vi "Net DC Global Gain Update.vi"(4 "Global Gain Correction":dbl, 5 "Device Trim List":string) -> (2 "Updated Trim List":string)   [LabVIEW 2010]
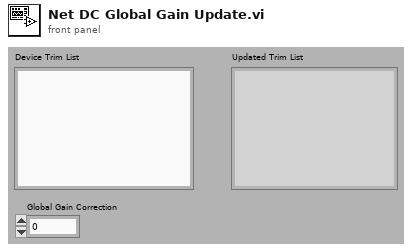
[diagram p1: front panel]
types:
  T1 = enum16{"U8", "U16", "U32", "U64", "I8", "I16", "I32", "I64"}
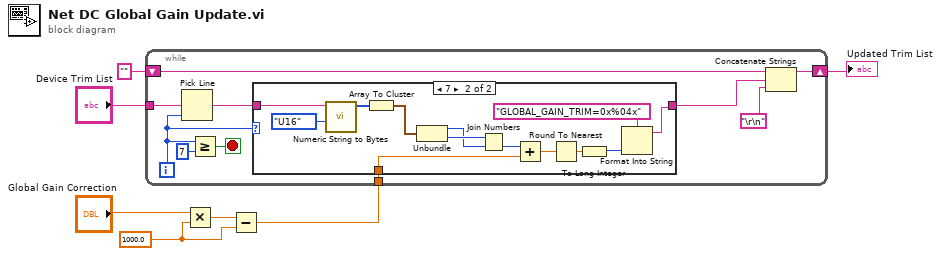
[diagram p0: block diagram]
diagram:
  w2 = 1000.0 ("y")
  n1 = Multiply(x="Global Gain Correction", y=w2) -> (x*y=w3:dbl)
  n2 = Subtract(x=w3, y=w2) -> (x-y=w1:dbl)
  n3 = while {
    tunnel: "Device Trim List" -> [w17]
    shift-right: [w15] -> w5
    shift-left: "" ("Device Trim List") -> [w14]
    tunnel: w1 -> [w8]
    i -> [w11]
    stop <- w12 stop-if-true
    n4 = Pick Line(multi-line string=w17, line index=w11) -> (output string=w10:string)  [unwired: 1 in]
    n5 = Greater Or Equal?(x=w11, y=7) -> (x >= y?=w12:bool)
    n6 = case shown="7" w11 {
      tunnel: [w18 w26] -> w9
      tunnel: w10 -> [w18 w31]
      tunnel: w8 -> [_ w20]
      frame 0, Default {
      }
      frame 7 {
        n7 = call "Numeric String to Bytes.vi"("Type"=T1."U16", "String"=w31) -> ("Byte Data"=w25:u8[])  [unwired: 8 in, 1 out]
        n8 = Array To Cluster(array=w25) -> (cluster=w24:cluster{"Byte Data[0]":u8, "Byte Data[1]":u8})
        n9 = Unbundle(w24) -> ("Byte Data[0]"=w22:u8, "Byte Data[1]"=w23:u8)
        n10 = Join Numbers(hi=w23, lo=w22) -> ((hi.lo)=w21:u16)
        n11 = Add(x=w21, y=w20) -> (x+y=w19:dbl)
        n12 = Round To Nearest(number=w19) -> (nearest integer value=w29:dbl)
        n13 = To Long Integer(number=w29) -> (32bit integer=w28:i32)
        n14 = Format Into String(format string="GLOBAL_GAIN_TRIM=0x%04x", w28) -> (resulting string=w26:string)  [unwired: 2 in, 1 out]
      }
    }
    n15 = Concatenate Strings(w14, w9, "\r\n") -> (w15:string)
  }
  "Updated Trim List" <- w5
